vi "Read ColumnSizes.vi"(8 "error in (no error)":errorcluster, 11 "AdjustableMulticolumnListbox in":refnum<class "AdjMCLB.lvclass">) -> (0 "error out":errorcluster, 2 "ColumnSizes":i32[](array[numeric]), 3 "AdjustableMulticolumnListbox out":refnum<class "AdjMCLB.lvclass">)   [LabVIEW 2020, in "AdjMCLB.lvclass"]
uses:
  AdjMCLB.lvclass
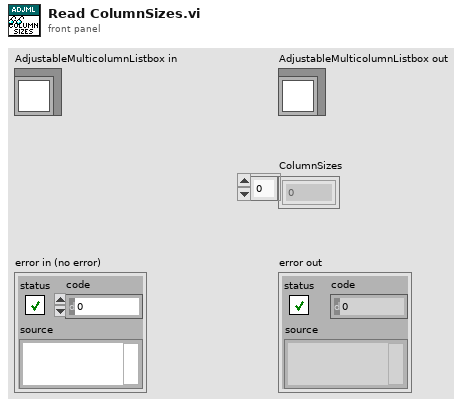
[diagram p1: front panel]
types:
  T1 = typedef "AdjustableMulticolumnListbox.lvclass/State Data.ctl" = cluster{"FitControlToPane?":bool, "ColumnSizes":i32[]}
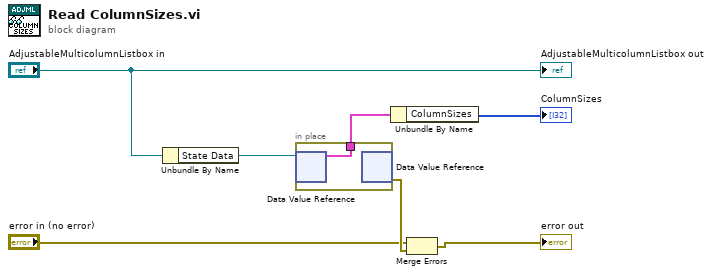
[diagram p0: block diagram]
diagram:
  n1 = Unbundle By Name("AdjustableMulticolumnListbox in") -> ("State Data"=w7:refnum<data-value>)
  n2 = in-place {
    in-place-border: [w8] -> w6
    n3 = in-place-dvr #1(w7) -> (w8:T1)  [unwired: 1 out]
    n4 = in-place-dvr #1() -> (w5:errorcluster)  [unwired: 1 in, 1 out]
  }
  n5 = Unbundle By Name(w6) -> ("ColumnSizes"=→"ColumnSizes":i32[])
  n6 = Merge Errors("error in (no error)", w5) -> (→"error out":errorcluster)
  "AdjustableMulticolumnListbox out" <- "AdjustableMulticolumnListbox in"
